vi "PWM Configure Port.vi"(8 "Error In":errorcluster, 11 "ChipKit Resource":T1={"COM Port"="", "Board Type"=enum."ChipKit uC32", "Connection Type"=enum."USB / Serial", "Baud Rate (115200)"=15, "Bytes Per Packet (15)"=15}) -> (0 "Error Out":errorcluster, 2 "PWM Pins":u8[](array[numeric])=[3, 5, 6], 3 "ChipKit Resource":T1={"COM Port"="", "Board Type"=enum."ChipKit uC32", "Connection Type"=enum."USB / Serial", "Baud Rate (115200)"=15, "Bytes Per Packet (15)"=15})   [LabVIEW 2011, in "LabVIEW Interface for ChipKit.lvlib"]
doc: "Configure 3 Arduino pins to use for PWM."
uses:
  LabVIEW Interface for ChipKit.lvlib
  Private/Type Defs/Pin Mode.ctl
  Private/Type Defs/Board Type.ctl
  Private/Type Defs/Chipkit Resource.ctl
  Private/Type Defs/Connection Type.ctl
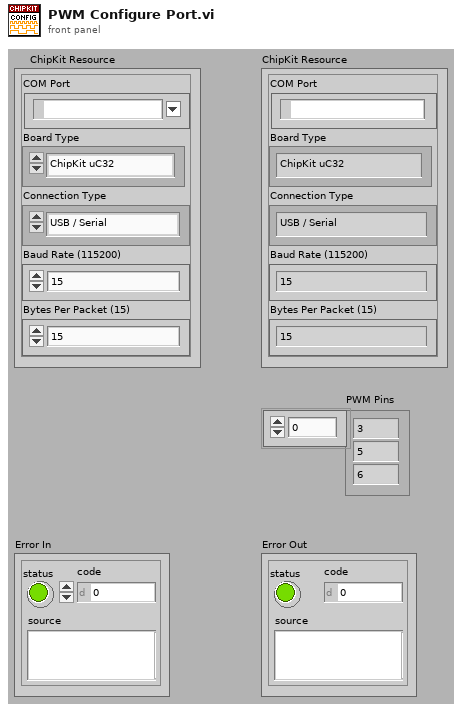
[diagram p1: front panel]
types:
  T1 = typedef "LabVIEW Interface for ChipKit.lvlib/Chipkit Resource.ctl" = cluster{"COM Port":refnum<visa-resource-name>, "Board Type":T2, "Connection Type":T3, "Baud Rate (115200)":u32, "Bytes Per Packet (15)":u32}
  T2 = typedef "LabVIEW Interface for ChipKit.lvlib/Board Type.ctl" = enum16{"ChipKit uC32", "ChipKit Uno32", "ChipKit Max32"}
  T3 = typedef "LabVIEW Interface for ChipKit.lvlib/Connection Type.ctl" = enum8{"USB / Serial", "XBEE", "BlueSmirf (Bluetooth)"}
  T4 = typedef "LabVIEW Interface for ChipKit.lvlib/Pin Mode.ctl" = enum16{"Input", "Output"}
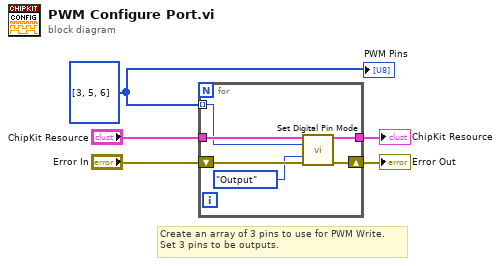
[diagram p0: block diagram]
diagram:
  w1 = u8[] [3, 5, 6]
  # "Create an array of 3 pins to use for PWM Write.\nSet 3 pins to be outputs."
  n1 = for {
    tunnel: "ChipKit Resource" -> [w11]
    tunnel: [w10] -> w4
    tunnel: w1 -> [w7] mode=indexing
    shift-right: [w8] -> w2
    shift-left: "Error In" -> [w9]
    n2 = call "Set Digital Pin Mode.vi"("Arduino Resource"=w11, "Digital I/O Pin"=w7, "Pin Mode (Input)"=Pin_Mode."Output" ("Pin Mode"), "error in"=w9) -> ("Arduino Resource"=w10:T1, "error out"=w8:errorcluster)  [unwired: 10 in]
  }
  "Error Out" <- w2
  "ChipKit Resource" <- w4
  "PWM Pins" <- w1
